vi "GetNavigations.vi"(11 "ButtonDefinitions":T1[](array[typedef])) -> (2 "Array":cluster{T1[]}[](array[cluster]), 3 "Navigations":string[](array[string]))   [LabVIEW 2021, in "ButtonBarFlow.lvlib"]
uses:
  ButtonBarFlow.lvlib
  TAFAOModule_GUI_VerticalButtonBar/VerticalButtonBar/ButtonCollection/ButtonDefinition.ctl
  TAFAOModule_GUI_VerticalButtonBar/VerticalButtonBar/ButtonCollection/ButtonCollection.lvclass
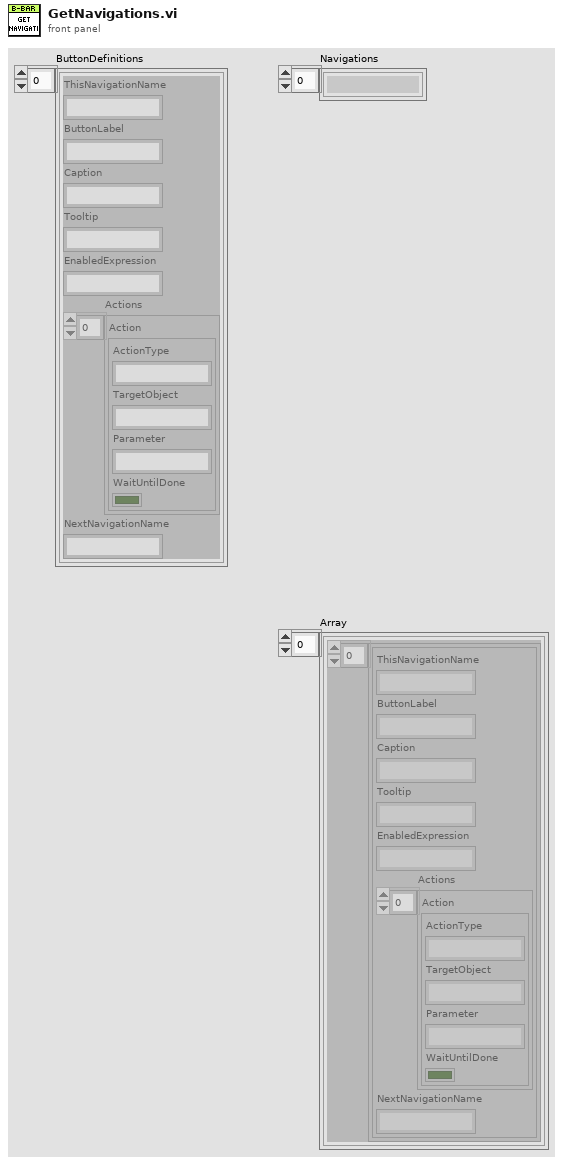
[diagram p1: front panel]
types:
  T1 = typedef "ButtonCollection.lvclass/ButtonDefinition.ctl" = cluster{"ThisNavigationName":string, "ButtonLabel":string, "Caption":string, "Tooltip":string, "EnabledExpression":string, "Actions":cluster{"ActionType":string, "TargetObject":string, "Parameter":string, "WaitUntilDone":bool}[], "NextNavigationName":string}
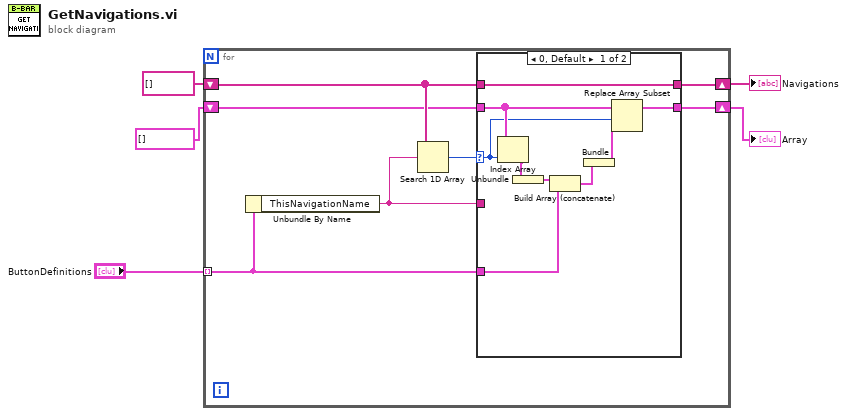
[diagram p0: block diagram]
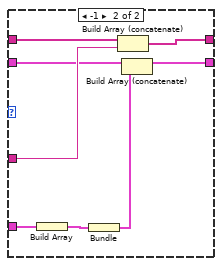
[diagram p2: hidden frame]
diagram:
  n1 = for {
    tunnel: "ButtonDefinitions" -> [w6] mode=indexing
    shift-right: [w9] -> w3
    shift-left: string[] [] -> [w11]
    shift-right: [w7] -> w4
    shift-left: cluster{T1[]}[] [] -> [w8]
    n2 = Unbundle By Name(w6) -> ("ThisNavigationName"=w10:string)
    n3 = Search 1D Array(1D array=w11, element=w10) -> (index of element=w12:i32)  [unwired: 1 in]
    n4 = case shown="0, Default" w12 {
      selector: w12 -> [w15 _]
      tunnel: [w21 w28] -> w9
      tunnel: w11 -> [w21 w29]
      tunnel: w10 -> [_ w27]
      tunnel: w8 -> [w16 w26]
      tunnel: [w17 w25] -> w7
      tunnel: w6 -> [w18 w24]
      frame 0, Default {
        n5 = Index Array(array=w16, index=w15) -> (element=w20:cluster{T1[]})
        n6 = Unbundle(w20) -> (w19:T1[])
        n7 = Build Array (concatenate)(w19, w18) -> (w13:T1[])
        n8 = Bundle(w13) -> (w14:cluster{T1[]})  [unwired: 1 in]
        n9 = Replace Array Subset(array=w16, new element=w14, index=w15) -> (w17:cluster{T1[]}[])
      }
      frame -1 {
        n10 = Build Array(w24) -> (w23:T1[])
        n11 = Bundle(w23) -> (w22:cluster{T1[]})  [unwired: 1 in]
        n12 = Build Array (concatenate)(w29, w27) -> (w28:string[])
        n13 = Build Array (concatenate)(w26, w22) -> (w25:cluster{T1[]}[])
      }
    }
  }
  "Array" <- w4
  "Navigations" <- w3
